vi "Emballage_BDD_Verif_TRAC_.vi"(8 "Error in":errorcluster caption="Error in (no error)", 11 "Param_produitPricipal":string[](array[string])) -> (0 "Error out":errorcluster, 3 "Param_produit OUT":string[](array[string]))   [LabVIEW 2018]
panel:
  out "sous-chaîne suivante":string
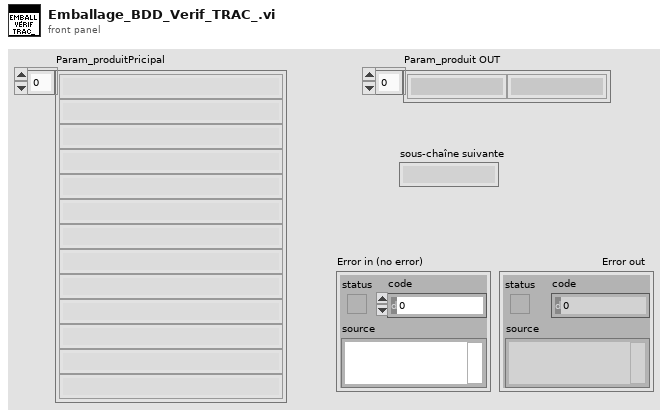
[diagram p1: front panel]
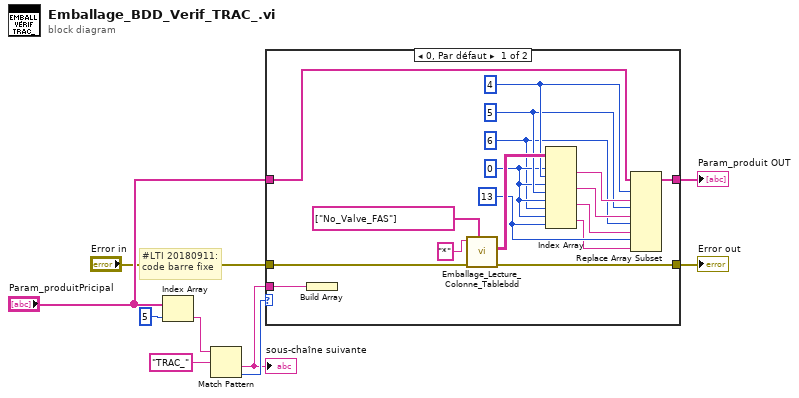
[diagram p0: block diagram]
diagram:
  # "#LTI 20180911:\ncode barre fixe"
  n1 = Index Array(array="Param_produitPricipal", index=5 ("indice")) -> (element=w8:string)
  n2 = Match Pattern(string=w8, regular expression="TRAC_" ("expression régulière")) -> (after substring=w3:string, offset past match=w6:i32)  [unwired: 1 in, 2 out]
  "sous-chaîne suivante" <- w3
  n3 = case shown="0, Par défaut" w6 {
    tunnel: "Param_produitPricipal" -> [w22 w28]
    tunnel: [w12 w28] -> w4
    tunnel: w3 -> [w24 _]
    tunnel: "Error in" -> [w11 w27]
    tunnel: [w10 w27] -> w1
    frame 0, Default {
      w14 = 13 ("indice")
      w15 = 6 ("indice")
      w19 = 5 ("indice")
      w21 = 4 ("indice")
      w17 = 0 ("indice (ligne)")
      n4 = Build Array(w24) -> ()  [unwired: 1 out]
      n5 = call "Emballage_Lecture_Colonne_Tablebdd.vi"("Where colonne"=string[] ["No_Valve_FAS"], "Error in"=w11, "Colonne"="*") -> ("Error out"=w10:errorcluster, "Result Set"=w23:string[][])  [unwired: 6 in, 1 out]
      n6 = Index Array(array=w23, index (row) #1=w17, index (col) #1=w21, index (row) #2=w17, index (col) #2=w19, index (row) #3=w17, index (col) #3=w15, index (row) #4=w17, index (col) #4=w14) -> (element #1=w20:string, element #2=w18:string, element #3=w16:string, element #4=w13:string)
      n7 = Replace Array Subset(array=w22, new element #1=w20, index #1=w21, new element #2=w18, index #2=w19, new element #3=w16, index #3=w15, new element #4=w13, index #4=w14) -> (w12:string[])
    }
    frame -1 {
    }
  }
  "Param_produit OUT" <- w4
  "Error out" <- w1
